vi "Untitled 1.vi"() -> ()   [LabVIEW 2009]
panel:
  out "Waveform Chart":dynamicdata(graph)
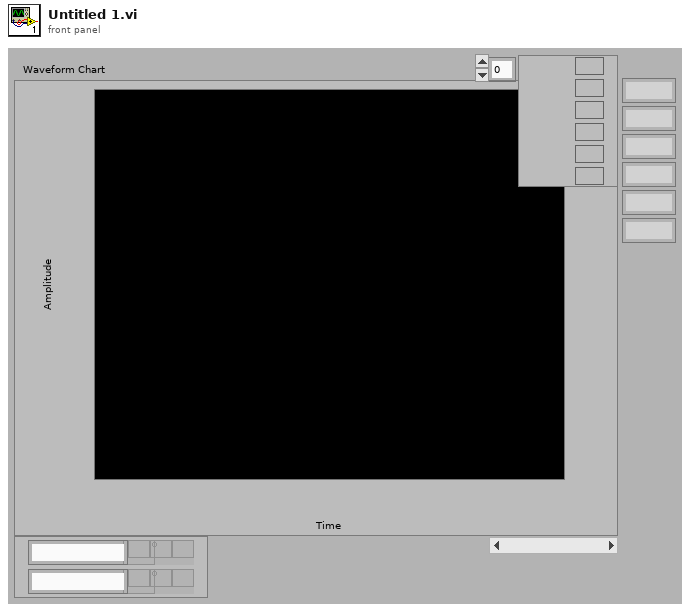
[diagram p1: front panel]
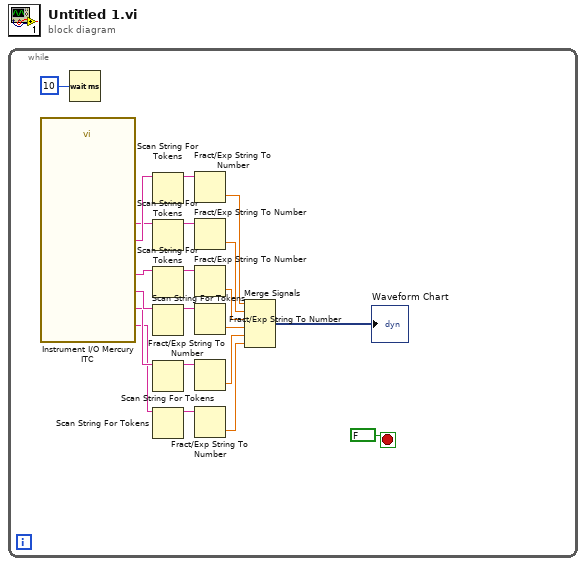
[diagram p0: block diagram]
diagram:
  n1 = while {
    stop <- FALSE stop-if-true
    n2 = call "Instrument I/O Mercury ITC"() -> ("CCS Res"=w7:string, "AB temp"=w10:string, "AB Res"=w11:string, "Cernox res"=w4:string, "Cernox temp"=w17:string, "CCS temp"=w21:string)  [unwired: 21 in, 1 out]
    n3 = Wait (ms)(milliseconds to wait=u32 10) -> ()  [unwired: 1 out]
    n4 = Scan String For Tokens(9:w21) -> (3:w20:string)  [unwired: 5 in, 3 out]
    n5 = Scan String For Tokens(9:w17) -> (3:w16:string)  [unwired: 5 in, 3 out]
    n6 = Scan String For Tokens(9:w11) -> (3:w13:string)  [unwired: 5 in, 3 out]
    n7 = Scan String For Tokens(9:w10) -> (3:w9:string)  [unwired: 5 in, 3 out]
    n8 = Scan String For Tokens(9:w7) -> (3:w6:string)  [unwired: 5 in, 3 out]
    n9 = Scan String For Tokens(9:w4) -> (3:w3:string)  [unwired: 5 in, 3 out]
    n10 = Fract/Exp String To Number(string=w20) -> (number=w15:dbl)  [unwired: 3 in, 1 out]
    n11 = Fract/Exp String To Number(string=w16) -> (number=w14:dbl)  [unwired: 3 in, 1 out]
    n12 = Fract/Exp String To Number(string=w13) -> (number=w12:dbl)  [unwired: 3 in, 1 out]
    n13 = Fract/Exp String To Number(string=w9) -> (number=w8:dbl)  [unwired: 3 in, 1 out]
    n14 = Fract/Exp String To Number(string=w6) -> (number=w5:dbl)  [unwired: 3 in, 1 out]
    n15 = Fract/Exp String To Number(string=w3) -> (number=w2:dbl)  [unwired: 3 in, 1 out]
    n16 = Merge Signals(w15, w14, w12, w8, w5, w2) -> (→"Waveform Chart":dynamicdata)
  }
